vi "Create VI Documentation.vi"(0 "VI Path":path, 1 "Library Examples Folder":path, 2 "Library Name":string, 5 "Template VI HTML Doc":path, 9 "Target Folder":path, 11 "error in (no error)":errorcluster, 12 "Example VIs":string[](array[string]), 14 "Supplimental VI Information":string="Use the dictionary reference when calling other <a href=\"Dictionary.html\">Dictionary</a> functions.") -> (3 "VI Description":string, 4 "HTML file path":path, 6 "VI Name":string, 15 "error out":errorcluster)   [LabVIEW 2011]
uses:
  Keyword Values - Cluster -.ctl
  <userlib>/_OpenG.lib/file/file.llb/Compare Two Paths - Scalar__ogtk.vi
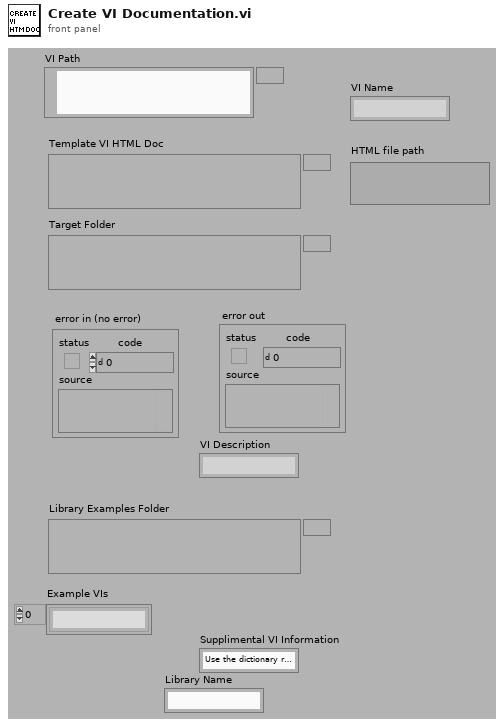
[diagram p1: front panel]
types:
  T1 = cluster{"VI Name":string, "Example VI Name":string, "Example VI Path":string, "Library Examples Folder":string, "Library Examples Folder Escaped":string, "Library Name":string}
  T2 = typedef "Keyword Values - Cluster -.ctl" = cluster{"VI Name":string, "VI Description":string, "VI ConPane Image Path":string, "Table of VI Parameters":string, "Supplimental VI Information":string, "Link to Additional VI Information and Examples":string, "Additional VI Information":string, "Example Information":string, "Library Examples Folder":string, "Library Name":string, "Library Examples Folder Escaped":string}
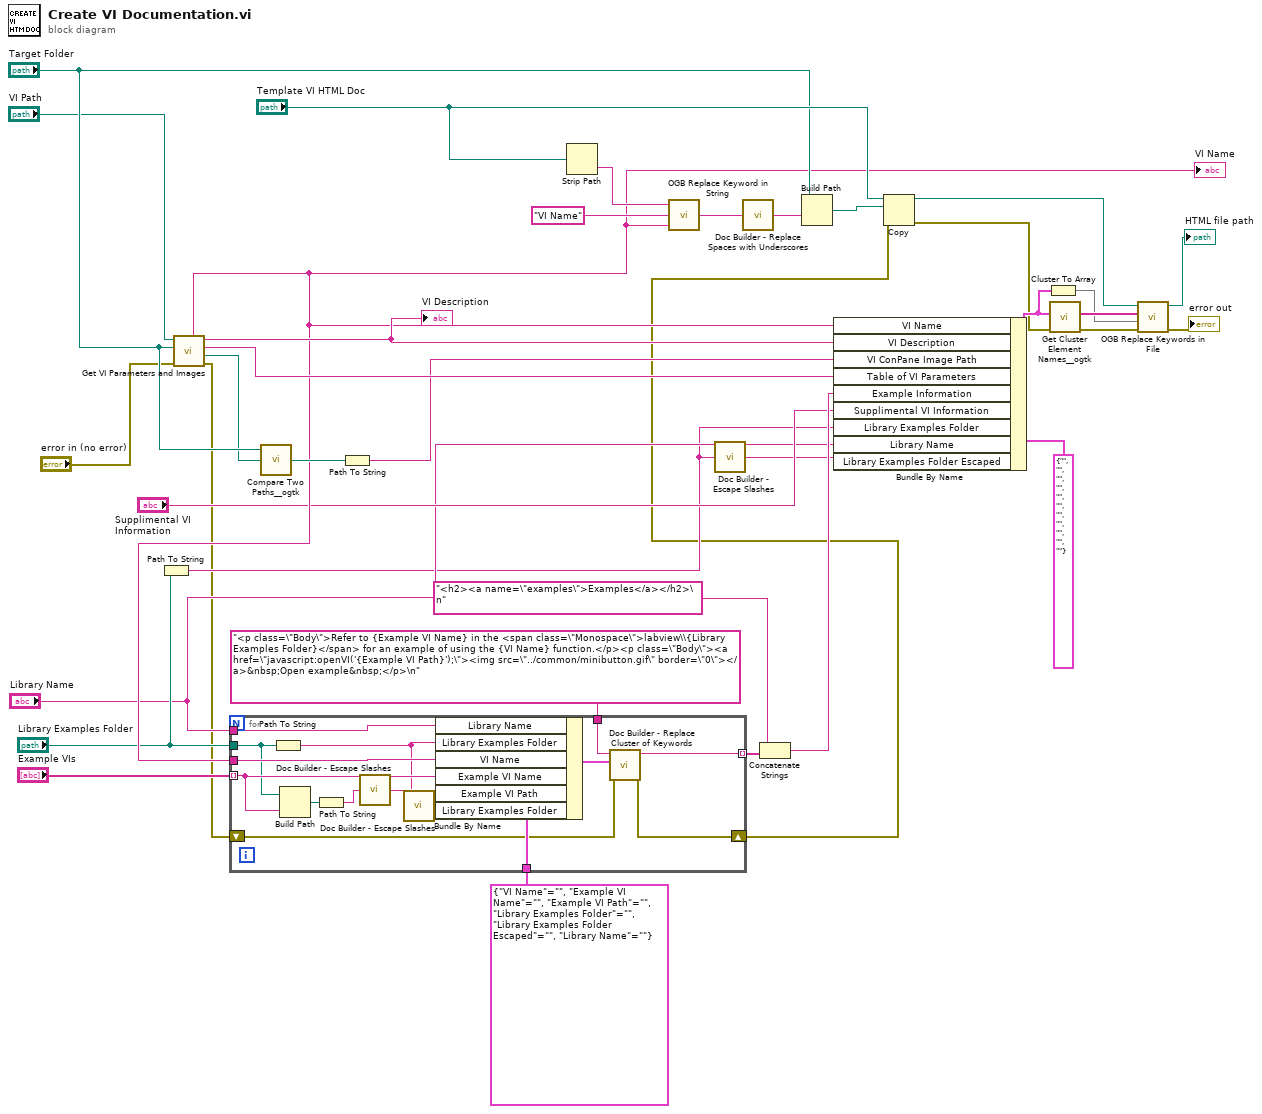
[diagram p0: block diagram]
diagram:
  n1 = Path To String(path="Library Examples Folder") -> (string=w3:string)
  n2 = call "Get VI Parameters and Images.vi"("error in (no error)"="error in (no error)", "Target Folder"="Target Folder", "VI Path"="VI Path") -> ("error out"=w2:errorcluster, "Icon Image Path"=w22:path, "String"=w27:string, "VI Description"=w28:string, "VI Name"=w13:string)  [unwired: 3 in, 1 out]
  "VI Name" <- w13
  "VI Description" <- w28
  n3 = for {
    tunnel: "<p class=\"Body\">Refer to {Example VI Name} in the <span class=\"Monospace\">labview\\{Library Examples Folder}</span> for an example of using the {VI Name} function.</p><p class=\"Body\"><a href=\"javascript:openVI('{Example VI Path}');\"><img src=\"../common/minibutton.gif\" border=\"0\"></a>&nbsp;Open example&nbsp;</p>\n" ("Keyword") -> [w52]
    tunnel: T1 {"VI Name"="", "Example VI Name"="", "Example VI Path"="", "Library Examples Folder"="", "Library Examples Folder Escaped"="", "Library Name"=""} -> [w51]
    tunnel: w13 -> [w49]
    tunnel: [w48] -> w12 mode=indexing
    tunnel: "Library Examples Folder" -> [w44]
    tunnel: "Example VIs" -> [w47] mode=indexing
    tunnel: "Library Name" -> [w40]
    shift-right: [w38] -> w1
    shift-left: w2 -> [w39]
    n4 = Path To String(path=w44) -> (string=w41:string)
    n5 = Build Path(base path=w44, name or relative path=w47) -> (appended path=w46:path)
    n6 = Path To String(path=w46) -> (string=w45:string)
    n7 = call "Doc Builder - Escape Slashes.vi"("String"=w45) -> ("String out"=w42:string)  [unwired: 4 in]
    n8 = call "Doc Builder - Escape Slashes.vi"("String"=w41) -> ("String out"=w43:string)  [unwired: 4 in]
    n9 = Bundle By Name(cluster=w51, "Library Name"=w40, "Library Examples Folder"=w41, "VI Name"=w49, "Example VI Name"=w47, "Example VI Path"=w42, "Library Examples Folder"=w43) -> (w50:T1)
    n10 = call "Doc Builder - Replace Cluster of Keywords.vi"("error in (no error)"=w39, "VCluster of KeyVals"=w50, "String"=w52) -> ("error out"=w38:errorcluster, "String out"=w48:string)  [unwired: 7 in]
  }
  n11 = call-poly <userlib>:"Compare Two Paths__ogtk.vi"("path2"=w22, "path1"="Target Folder") -> ("relative path from 1 to 2"=w21:path)  [unwired: 1 in, 2 out]
  n12 = Path To String(path=w21) -> (string=w20:string)
  n13 = Strip Path(path="Template VI HTML Doc") -> (name=w37:string)  [unwired: 1 out]
  n14 = call "OGB Replace Keyword in String.vi"("Value"=w13, "Keyword"="VI Name", "String"=w37) -> ("String out"=w18:string)
  n15 = call "Doc Builder - Escape Slashes.vi"("String"=w3) -> ("String out"=w5:string)  [unwired: 4 in]
  n16 = call "Doc Builder - Replace Spaces with Underscores.vi"("String"=w18) -> ("String out"=w17:string)  [unwired: 4 in]
  n17 = Concatenate Strings("<h2><a name=\"examples\">Examples</a></h2>\n" ("Keyword"), w12) -> (w10:string)
  n18 = Build Path(base path="Target Folder", name or relative path=w17) -> (appended path=w34:path)
  n19 = Bundle By Name(cluster=T2 {"VI Name"="", "VI Description"="", "VI ConPane Image Path"="", "Table of VI Parameters"="", "Supplimental VI Information"="", "Link to Additional VI Information and Examples"="", "Additional VI Information"="", "Example Information"="", "Library Examples Folder"="", "Library Name"="", "Library Examples Folder Escaped"=""} ("Keyword Values"), "VI Name"=w13, "VI Description"=w28, "VI ConPane Image Path"=w20, "Table of VI Parameters"=w27, "Example Information"=w10, "Supplimental VI Information"="Supplimental VI Information", "Library Examples Folder"=w3, "Library Name"="Library Name", "Library Examples Folder Escaped"=w5) -> (w30:T2)
  n20 = Copy(8:w1, 10:w34, 11:"Template VI HTML Doc") -> (0:w24:errorcluster, 3:w33:path)  [unwired: 2 in, 1 out]
  n21 = Cluster To Array(cluster=w30) -> (array=w31:string[])
  n22 = call <userlib>:"Get Cluster Element Names__ogtk.vi"("error in (no error)"=w24, "Cluster"=w30) -> ("error out"=w25:errorcluster, "Element Names"=w32:string[])  [unwired: 8 in]
  n23 = call "OGB Replace Keywords in File.vi"("error in (no error)"=w25, "Values"=w31, "Keywords"=w32, "file path"=w33) -> ("error out"=→"error out":errorcluster, "dup file path"=→"HTML file path":path)  [unwired: 6 in]
